vi "Populate Ctrl.vi"(8 "error in (no error)":errorcluster, 11 "Field Interface in":refnum<class "Field Interface.lvclass">) -> (0 "error out":errorcluster, 3 "Field Interface out":refnum<class "Field Interface.lvclass">)   [LabVIEW 2020, in "Field Interfaces.lvlib" / "Field Interface.lvclass"]
uses:
  Field Interface.lvclass
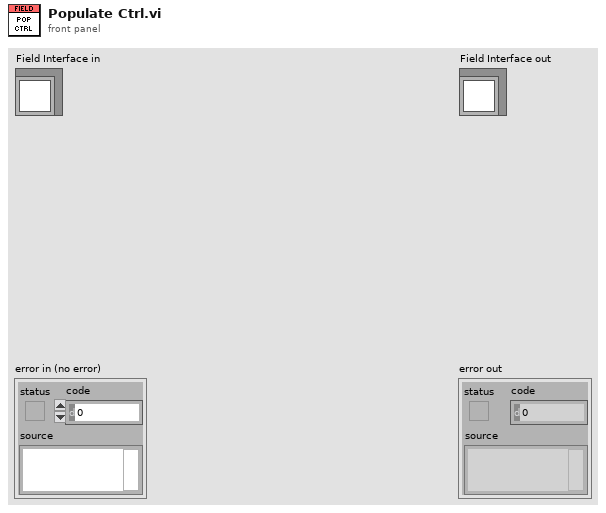
[diagram p1: front panel]
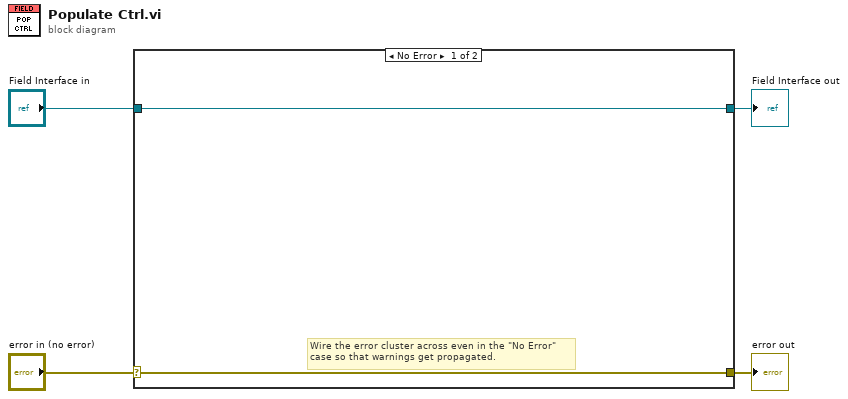
[diagram p0: block diagram]
diagram:
  n1 = case shown="No Error" "error in (no error)" {
    selector: "error in (no error)" -> [w5 w8]
    tunnel: [w5 w8] -> w3
    tunnel: [w6 w7] -> w1
    tunnel: "Field Interface in" -> [w6 w7]
    frame No Error {
      # "Wire the error cluster across even in the \"No Error\"\ncase so that warnings get propagated."
    }
    frame Error {
    }
  }
  "error out" <- w3
  "Field Interface out" <- w1
